vi "PSK_Packet_Mod.vi"(11 "user base bit pattern":i8[](array[numeric]) caption="Input bit stream") -> (3 "output complex waveform":T1 {"Y" format="%.3f"; "dt" format="%^.2e"; "t0" format="%.4f"})   [LabVIEW 2014]
uses:
  <vilib>/addons/Modulation/Analog/controls/Complex Data Waveform.ctl
  <vilib>/addons/Modulation/Digital/General/MT Generate Bits (Galois, PN Order).vi
  <vilib>/addons/Modulation/Digital/Support/Common/Validators/mod_Generate Bits Validate.vi
  <vilib>/addons/Modulation/Analog/support/mod_Set Error Source.vi
  <vilib>/addons/Modulation/Digital/General/MT Generate PSK System Parameters(M).vi
  <vilib>/addons/Modulation/Digital/Support/Common/Validators/mod_Generate Filter Coefficients Validate.vi
  <vilib>/addons/Modulation/Digital/General/subVIs/mod_Generate Filter Coefficients.vi
  <vilib>/addons/Modulation/Digital/General/subVIs/mod_Generate Bits PN Sequence.vi
  <vilib>/addons/Modulation/Digital/General/MT Generate Bits (User Defined).vi
  <vilib>/addons/Modulation/niDMT.lvlib
  <vilib>/addons/Modulation/niAMT.lvlib
panel:
  out "bits sent":i32
  out "input bit stream":i8[](array[numeric]) caption="output bit stream"
  in  "IQ Sampling\nRate [S/sec]":dbl=500000.0 format="%#.6p"
  in  "filter parameters":T2={"Alpha"=0.5, "Filter Length"=6, "TX Filter"=enum."Root Raised Cos"} {"Alpha" format="%.2f"}
  in  "QPSK System Parameters":T3={"Samples per Symbol"=8, "symbol map"=[], "Differential PSK"=enum."disable", "PSK type"=0} {"PSK type" items=["normal", "shifted", "offset"]; "symbol map" format="%.3f"}
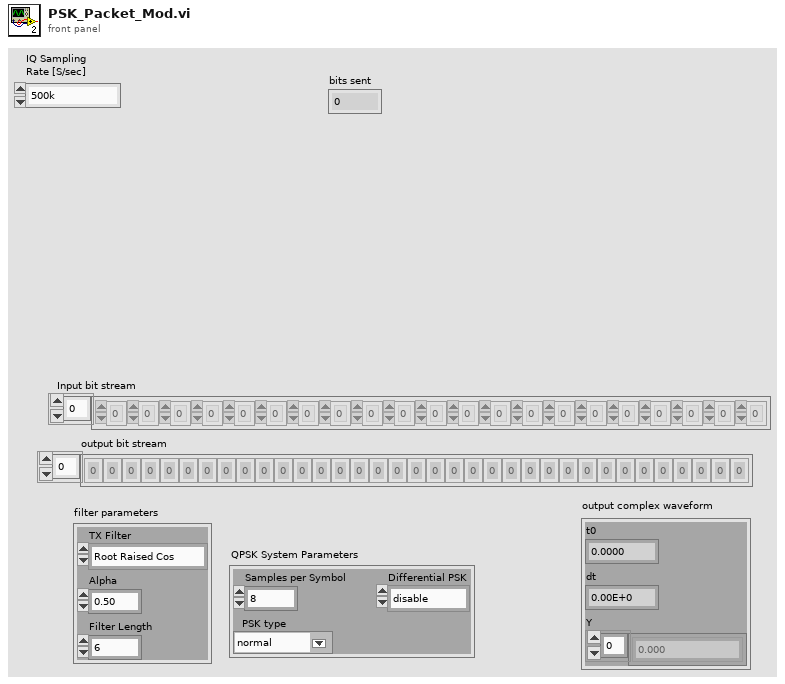
[diagram p1: front panel]
types:
  T1 = typedef "niAMT.lvlib/Complex Data Waveform.ctl" = cluster{"t0":dbl, "dt":dbl, "Y":cdb[]}
  T2 = cluster{"Alpha":dbl, "Filter Length":i32, "TX Filter":enum16{"none", "Raised Cosine", "Root Raised Cos", "Gaussian"}}
  T3 = cluster{"Samples per Symbol":i32, "symbol map":cdb[], "Differential PSK":enum16{"disable", "enable"}, "PSK type":u16}
  T4 = enum16{"FSK", "PSK", "QAM", "MSK", "PAM", "ASK", "CPM"}
  T5 = enum16{"none", "Raised Cosine", "Root Raised Cos", "Gaussian"}
  T6 = cluster{"samples per symbol (16)":i32, "symbol map":cdb[], "differential PSK":enum16{"disable", "enable"}, "PSK type":u16}
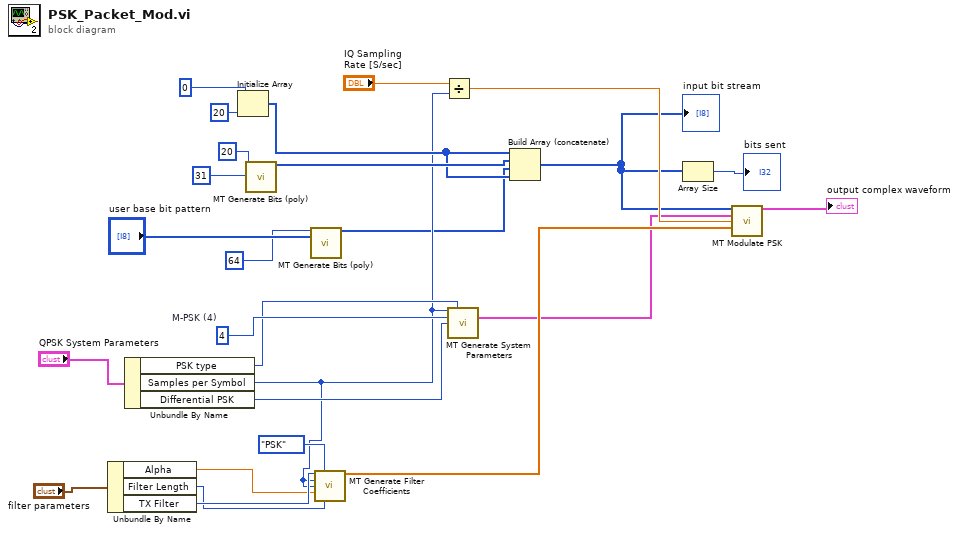
[diagram p0: block diagram]
diagram:
  w24 = 4  # M-PSK (4)
  n1 = Unbundle By Name("filter parameters") -> ("Alpha"=w20:dbl, "Filter Length"=w21:i32, "TX Filter"=w22:T5)
  n2 = Unbundle By Name("QPSK System Parameters") -> ("PSK type"=w23:u16, "Samples per Symbol"=w5:i32, "Differential PSK"=w25:enum16{"disable", "enable"})
  n3 = Initialize Array(i8 0 ("element"), 20 ("dimension size")) -> (w6:i8[])
  n4 = call-poly <vilib>:"MT Generate Bits (poly).vi"("total bits (128)"=20, "PN sequence order (9)"=31) -> ("output bit stream"=w7:i8[])  [unwired: 11 in, 2 out]
  n5 = call-poly <vilib>:"MT Generate Bits (poly).vi"("total bits (128)"=64, "user base bit pattern"="user base bit pattern") -> ("output bit stream"=w3:i8[])  [unwired: 12 in, 1 out]
  n6 = call <vilib>:"MT Generate Filter Coefficients.vi"("pulse shaping filter (none)"=w22, "modulation type"=T4."PSK", "pulse shaping samples per symbol (16)"=w5, "matched samples per symbol (16)"=w5, "filter parameter"=w20, "filter length (symbols)"=w21) -> ("pulse shaping filter coefficients"=w17:dbl[])  [unwired: 7 in, 2 out]
  n7 = Divide(x="IQ Sampling\nRate [S/sec]", y=w5) -> (x/y=w16:dbl)
  n8 = call-poly <vilib>:"MT Generate System Parameters.vi"("samples per symbol (16)"=w5, "PSK type"=w23, "M-PSK (4)"=w24, "differential PSK"=w25) -> ("PSK system parameters"=w4:T6)  [unwired: 9 in, 2 out]
  n9 = Build Array (concatenate)(w6, w7, w3, w6) -> (w13:i8[])
  "input bit stream" <- w13
  n10 = Array Size(array=w13) -> (size(s)=→"bits sent":i32)
  n11 = call <vilib>:"MT Modulate PSK.vi"("input bit stream"=w13, "PSK system parameters"=w4, "symbol rate (Hz)"=w16, "pulse shaping filter coefficients"=w17) -> ("output complex waveform"=→"output complex waveform":T1)  [unwired: 9 in, 2 out]
